vi "Get_Pulse.vi"(2 "error in":errorcluster, 3 "Filename (.ini)":string="Config_Ver_1\\pulse_sequence.ini") -> (0 "error out":errorcluster, 1 "Pulse sequence":T1[](array[typedef]) {"channel" min=2 max=13 step=1})   [LabVIEW 2021]
uses:
  Drivers/Arduino_Pulse_Generator/Configurate/Channel_Pulse_Stream.ctl
  <vilib>/Utility/config.llb/Read Key (String).vi
  <vilib>/Utility/config.llb/NI_LVConfig.lvlib
panel:
  # "Remember that config files are .ini, \nconfig file will be save in ...\\Config_Files\\(filename).ini"
  # "One can easily add files into folder placed inside ...\\Config_Files\\ (folder)\nby writing Filename as (folder)\\(filename).ini, but firstly one have to manualy\ncreate that folder"
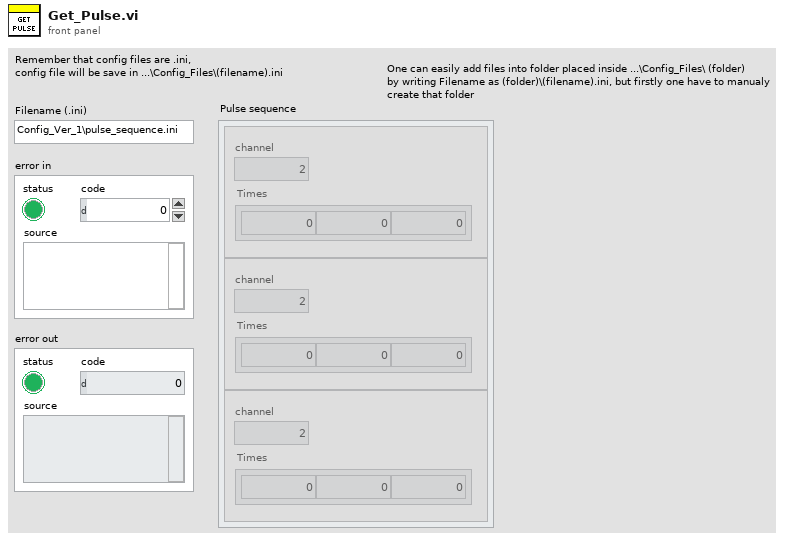
[diagram p1: front panel]
types:
  T1 = typedef "Channel_Pulse_Stream.ctl" = cluster{"Times":dbl[], "channel":u8}
  T2 = typedef "NI_LVConfig.lvlib/Config Data RefNum.ctl" = refnum<k1>
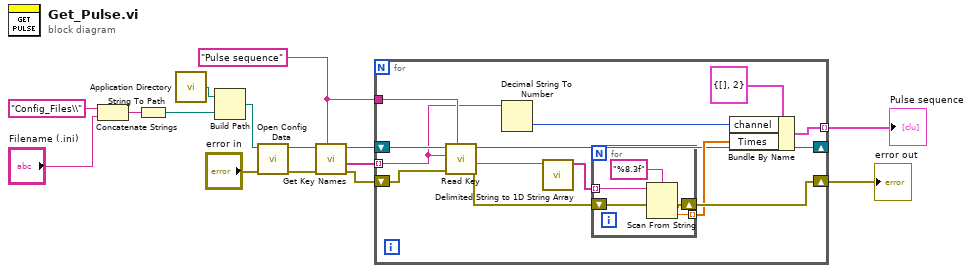
[diagram p0: block diagram]
diagram:
  w3 = "Pulse sequence" ("section")
  n1 = Concatenate Strings("Config_Files\\" ("string"), "Filename (.ini)") -> (w8:string)
  n2 = String To Path(string=w8) -> (path=w12:path)
  n3 = call <vilib>:"Application Directory.vi"() -> ("Application Directory"=w15:path)
  n4 = Build Path(base path=w15, name or relative path=w12) -> (appended path=w14:path)
  n5 = call <vilib>:"Open Config Data.vi"("error in (no error)"="error in", "configuration file path"=w14) -> ("error out"=w7:errorcluster, "refnum"=w11:T2)  [unwired: 7 in, 1 out]
  n6 = call <vilib>:"Get Key Names.vi"("section"=w3, "error in (no error)"=w7, "refnum"=w11) -> ("error out"=w5:errorcluster, "key names"=w6:string[], "refnum out"=w4:T2)  [unwired: 5 in, 1 out]
  n7 = for {
    tunnel: w6 -> [w16] mode=indexing
    shift-right: [w17] -> _
    shift-left: w4 -> [w28]
    shift-right: [w20] -> w1
    shift-left: w5 -> [w27]
    tunnel: w3 -> [w26]
    tunnel: [w18] -> w2 mode=indexing
    n8 = call-poly <vilib>:"Read Key.vi"("section"=w26, "error in (no error)"=w27, "key"=w16, "refnum"=w28) -> ("error out"=w21:errorcluster, "value"=w23:string, "refnum out"=w17:T2)  [unwired: 4 in, 1 out]
    n9 = Decimal String To Number(string=w16) -> (number=w24:i32)  [unwired: 2 in, 1 out]
    n10 = call <vilib>:"Delimited String to 1D String Array.vi"("delimited string"=w23) -> ("string array"=w22:string[])  [unwired: 10 in]
    n11 = for {
      tunnel: w22 -> [w33] mode=indexing
      tunnel: [w31] -> w19 mode=indexing
      shift-right: [w30] -> w20
      shift-left: w21 -> [w29]
      n12 = Scan From String(format string="%8.3f", input string=w33, error in=w29) -> (error out=w30:errorcluster, output 1=w31:dbl)  [unwired: 2 in, 2 out]
    }
    n13 = Bundle By Name(cluster=T1 {"Times"=[], "channel"=2} ("Channel pulse stream"), "channel"=w24, "Times"=w19) -> (w18:T1)
  }
  "Pulse sequence" <- w2
  "error out" <- w1
